vi "数据输入.vi"() -> ()   [LabVIEW 2018]
panel:
  in  "字符串":string
  in  "数值":dbl
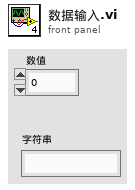
[diagram p1: front panel]
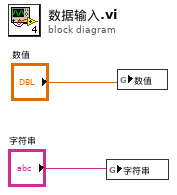
[diagram p0: block diagram]
diagram:
  n1 = global write "全局变量.vi" "字符串"("字符串") -> ()
  n2 = global write "全局变量.vi" "数值"("数值") -> ()
